vi "RH vector map_two devices_BF_LD-400_MFLI_MF-MD_PK_V5.0.vi"() -> ()   [LabVIEW 2016]
uses:
  Labview Drivers/MFLI/LabOneLabVIEW-19.05.64471/LabOneLabVIEW-19.05.64471/Zurich Instruments LabOne/Public/Configure/ziGetValueDemodSampleEx.vi
  Labview Drivers/MFLI/LabOneLabVIEW-19.05.64471/LabOneLabVIEW-19.05.64471/Zurich Instruments LabOne/Zurich Instruments LabOne.lvlib
panel:
  in  "Number average":i32=50
  out "Sweeping Magnetic Field (T)":dbl=3.018e-06 format="%#_13g"
  in  "Sweeping Magnet ramp rate (T/min)":string="0.03"
  in  "Sweeping Magnet IP Address":string="169.254.239.127"
  in  "Sweeping Magnet stabilization time (s)":dbl=1.0
  in  "From 1":dbl[](array[numeric])=[0.0] min=-3000.0 max=3000.0 format="%.1e"
  in  "To 1":dbl[](array[numeric])=[7.0] min=-3000.0 max=3000.0 format="%.1e"
  in  "Step 1":dbl[](array[numeric])=[0.05] min=-3000.0 max=3000.0 format="%.1e"
  in  "Stable Magnet stabilization time (s)":dbl=2.0 format="%#_13g"
  in  "Stable Magnet ramp rate (T/min)":string="0.03"
  out "data 2":dbl[](array[numeric])=[-1.3078e-05, 151.2, -2.85209836e-06, 4.947488930549757e-09, 8.074867339038734e-08, 16.321142810806588, -0.15000000000000074, -1.5000000000000073e-07]
  in  "Tab Control":enum32{"Device 1", "Device 2"}(tab)
  out "Rx vs H sweep (Device 1)":cluster{dbl, "Field Reading":dbl}[](graph)=[{1e-05, "Field Reading"=161.35840446232214}, {9.9e-06, "Field Reading"=41.860127097564245}, {9.800000000000001e-06, "Field Reading"=32.841407973882895}, {9.7e-06, "Field Reading"=32.83190215267119}, {9.600000000000001e-06, "Field Reading"=43.61342880349138}, {9.500000000000002e-06, "Field Reading"=37.97014058703433}, {9.400000000000001e-06, "Field Reading"=38.51287388600995}, {9.300000000000002e-06, "Field Reading"=35.71104185616921}, {9.200000000000003e-06, "Field Reading"=27.88224302316775}, {9.100000000000003e-06, "Field Reading"=31.112497747096224}, {9.000000000000004e-06, "Field Reading"=43.297646700361845}, {8.900000000000005e-06, "Field Reading"=40.66271846445741}, {8.800000000000004e-06, "Field Reading"=29.818940517533726}, {8.700000000000005e-06, "Field Reading"=31.775513272715916}, {8.600000000000006e-06, "Field Reading"=37.91978142458641}, {8.500000000000005e-06, "Field Reading"=36.71319882227341}, {8.400000000000006e-06, "Field Reading"=31.958807556261263}, {8.300000000000005e-06, "Field Reading"=43.39712342184189}, {8.200000000000006e-06, "Field Reading"=32.202863280072044}, {8.100000000000007e-06, "Field Reading"=36.33973788345392}, {8.000000000000006e-06, "Field Reading"=39.998122128750744}, {7.900000000000007e-06, "Field Reading"=42.39197863784701}, {7.800000000000008e-06, "Field Reading"=36.855072728087}, {7.700000000000008e-06, "Field Reading"=37.128132172992295}, {7.6000000000000085e-06, "Field Reading"=39.17166376756487}, {7.500000000000009e-06, "Field Reading"=39.80265360388928}, {7.40000000000001e-06, "Field Reading"=35.051759054439025}, {7.30000000000001e-06, "Field Reading"=39.481888206274185}, {7.20000000000001e-06, "Field Reading"=32.72055016297702}, {7.10000000000001e-06, "Field Reading"=28.557051745816146}, {7.000000000000011e-06, "Field Reading"=43.331293404541874}, {6.900000000000011e-06, "Field Reading"=35.81893185166727}, {6.800000000000011e-06, "Field Reading"=35.072778559533276}, {6.700000000000012e-06, "Field Reading"=35.44203632589805}, {6.600000000000012e-06, "Field Reading"=42.36422061997487}, {6.500000000000012e-06, "Field Reading"=42.01793319760923}, {6.400000000000012e-06, "Field Reading"=39.81979223345381}, {6.300000000000013e-06, "Field Reading"=45.67249265404195}, {6.2000000000000135e-06, "Field Reading"=39.54411342959387}, {6.100000000000014e-06, "Field Reading"=40.504490195623234}, {6.0000000000000146e-06, "Field Reading"=41.75691081353343}, {5.900000000000015e-06, "Field Reading"=41.452122749226305}, {5.800000000000015e-06, "Field Reading"=32.38970051842595}, {5.700000000000015e-06, "Field Reading"=43.00244438430981}, {5.600000000000016e-06, "Field Reading"=51.65721457657372}, {5.500000000000016e-06, "Field Reading"=45.63355271030433}, {5.400000000000016e-06, "Field Reading"=45.93782542419175}, {5.300000000000017e-06, "Field Reading"=45.55193121698807}, {5.200000000000017e-06, "Field Reading"=49.74200540752808}, {5.100000000000017e-06, "Field Reading"=48.779849266236944}, {5.000000000000017e-06, "Field Reading"=55.987007769383574}, {4.900000000000018e-06, "Field Reading"=49.48719028405444}, {4.800000000000018e-06, "Field Reading"=41.40308707863719}, {4.7000000000000185e-06, "Field Reading"=53.784373814286994}, {4.6000000000000195e-06, "Field Reading"=44.085575612549306}, {4.50000000000002e-06, "Field Reading"=49.718341348618466}, {4.40000000000002e-06, "Field Reading"=53.65171728330762}, {4.300000000000021e-06, "Field Reading"=59.641548125735824}, {4.200000000000021e-06, "Field Reading"=47.06243760711321}, {4.100000000000021e-06, "Field Reading"=55.39894693411911}, {4.000000000000021e-06, "Field Reading"=62.51571936174172}, {3.900000000000021e-06, "Field Reading"=68.9035008907534}, {3.8000000000000212e-06, "Field Reading"=63.99606775314202}, {3.700000000000021e-06, "Field Reading"=66.77234365785664}, {3.600000000000021e-06, "Field Reading"=69.5179299545508}, {3.5000000000000207e-06, "Field Reading"=62.954254580455874}, {3.400000000000021e-06, "Field Reading"=73.81293930429145}, {3.3000000000000205e-06, "Field Reading"=70.82103242823298}, {3.2000000000000206e-06, "Field Reading"=69.76720206210479}, {3.1000000000000207e-06, "Field Reading"=78.80471547799624}, {3.0000000000000204e-06, "Field Reading"=67.44386101206055}, {2.9000000000000205e-06, "Field Reading"=82.59912131166654}, {2.80000000000002e-06, "Field Reading"=81.12168427698563}, {2.7000000000000203e-06, "Field Reading"=81.13823856191323}, {2.60000000000002e-06, "Field Reading"=84.63690509367076}, {2.50000000000002e-06, "Field Reading"=83.00020269365744}, {2.40000000000002e-06, "Field Reading"=93.0262013428328}, {2.30000000000002e-06, "Field Reading"=91.86498911211211}, {2.2000000000000196e-06, "Field Reading"=95.78189064219018}, {2.1000000000000197e-06, "Field Reading"=97.67903895306458}, {2.0000000000000194e-06, "Field Reading"=106.0177258797565}, {1.9000000000000195e-06, "Field Reading"=112.14543741308948}, {1.8000000000000194e-06, "Field Reading"=117.94072002587943}, {1.7000000000000193e-06, "Field Reading"=128.50868647129005}, {1.6000000000000192e-06, "Field Reading"=130.73283750941107}, {1.500000000000019e-06, "Field Reading"=131.1900544205175}, {1.400000000000019e-06, "Field Reading"=136.76914635961774}, {1.3000000000000189e-06, "Field Reading"=146.35130253331926}, {1.2000000000000188e-06, "Field Reading"=159.2235400585063}, {1.1000000000000187e-06, "Field Reading"=162.39683572656568}, {1.0000000000000186e-06, "Field Reading"=183.24820207539153}, {9.000000000000187e-07, "Field Reading"=198.59616773730164}, {8.000000000000187e-07, "Field Reading"=202.29711475013792}, {7.000000000000187e-07, "Field Reading"=229.13939118910707}, {6.000000000000187e-07, "Field Reading"=352.4121711509943}, {5.000000000000187e-07, "Field Reading"=497.13445785563255}, {4.000000000000188e-07, "Field Reading"=969.1807249612372}, {3.0000000000001883e-07, "Field Reading"=2319.3065167116256}, {2.000000000000188e-07, "Field Reading"=349.016889238513}, {1.000000000000188e-07, "Field Reading"=25.587807905491125}, {1.8790524691780774e-20, "Field Reading"=15.950426066262958}, {-9.999999999998122e-08, "Field Reading"=14.841961476733772}, {-1.9999999999998122e-07, "Field Reading"=11.215795144009844}, {-2.9999999999998125e-07, "Field Reading"=8.869104703440923}, {-3.9999999999998124e-07, "Field Reading"=16.959841129659424}, {-4.999999999999812e-07, "Field Reading"=9.789433803826673}, {-5.999999999999812e-07, "Field Reading"=15.811405982830719}, {-6.999999999999812e-07, "Field Reading"=13.778561448799387}, {-7.999999999999812e-07, "Field Reading"=17.07939251134803}, {-8.999999999999811e-07, "Field Reading"=11.567482110630706}, {-9.999999999999811e-07, "Field Reading"=17.189724606732675}, {-1.0999999999999812e-06, "Field Reading"=8.534332836325326}, {-1.1999999999999813e-06, "Field Reading"=9.679059096554875}, {-1.2999999999999814e-06, "Field Reading"=19.417316586661677}, {-1.3999999999999815e-06, "Field Reading"=12.522271815596387}, {-1.4999999999999816e-06, "Field Reading"=10.165331935185511}, {-1.5999999999999817e-06, "Field Reading"=15.941613676936976}]
  out "Ix 1 (A)":dbl=1.9993378263160822e-08
  out "Vx 1 (V)":dbl=3.18726712368179e-07
  out "Rx 1 (ohm)":dbl=15.941613676936976
  in  "MFLI Device 1 Address":string="DEV4382"
  in  "File Name Device 1":string="037_S4.5_NBVJ02_dVdImapping(Bz)_I18_R45_ac20nA(7.919Hz)_dcpre1_range0.2_step1.5m"
  out "Vy 1 (V)":dbl format="%#_13g"
  out "Iy 1 (A)":dbl format="%#_13g"
  in  "Folder":path=path "D:/Heng/Nb3Br8_JJ/Sb.3_NBVJ01"
  in  "MFLI Device 2 Address":string="DEV4496"
  in  "File Name Device 2":string="037_Sb.3_NBVJ01_dVdI_mapping(Bz)_I16_R34_ac5nA(13.3337Hz)_dcpre1_range0.2_step1.5m"
  out "Rx vs H sweep (Device 2)":cluster{dbl, "Field Reading":dbl}[](graph)=[{1e-05, "Field Reading"=161.35840446232214}, {9.9e-06, "Field Reading"=41.860127097564245}, {9.800000000000001e-06, "Field Reading"=32.841407973882895}, {9.7e-06, "Field Reading"=32.83190215267119}, {9.600000000000001e-06, "Field Reading"=43.61342880349138}, {9.500000000000002e-06, "Field Reading"=37.97014058703433}, {9.400000000000001e-06, "Field Reading"=38.51287388600995}, {9.300000000000002e-06, "Field Reading"=35.71104185616921}, {9.200000000000003e-06, "Field Reading"=27.88224302316775}, {9.100000000000003e-06, "Field Reading"=31.112497747096224}, {9.000000000000004e-06, "Field Reading"=43.297646700361845}, {8.900000000000005e-06, "Field Reading"=40.66271846445741}, {8.800000000000004e-06, "Field Reading"=29.818940517533726}, {8.700000000000005e-06, "Field Reading"=31.775513272715916}, {8.600000000000006e-06, "Field Reading"=37.91978142458641}, {8.500000000000005e-06, "Field Reading"=36.71319882227341}, {8.400000000000006e-06, "Field Reading"=31.958807556261263}, {8.300000000000005e-06, "Field Reading"=43.39712342184189}, {8.200000000000006e-06, "Field Reading"=32.202863280072044}, {8.100000000000007e-06, "Field Reading"=36.33973788345392}, {8.000000000000006e-06, "Field Reading"=39.998122128750744}, {7.900000000000007e-06, "Field Reading"=42.39197863784701}, {7.800000000000008e-06, "Field Reading"=36.855072728087}, {7.700000000000008e-06, "Field Reading"=37.128132172992295}, {7.6000000000000085e-06, "Field Reading"=39.17166376756487}, {7.500000000000009e-06, "Field Reading"=39.80265360388928}, {7.40000000000001e-06, "Field Reading"=35.051759054439025}, {7.30000000000001e-06, "Field Reading"=39.481888206274185}, {7.20000000000001e-06, "Field Reading"=32.72055016297702}, {7.10000000000001e-06, "Field Reading"=28.557051745816146}, {7.000000000000011e-06, "Field Reading"=43.331293404541874}, {6.900000000000011e-06, "Field Reading"=35.81893185166727}, {6.800000000000011e-06, "Field Reading"=35.072778559533276}, {6.700000000000012e-06, "Field Reading"=35.44203632589805}, {6.600000000000012e-06, "Field Reading"=42.36422061997487}, {6.500000000000012e-06, "Field Reading"=42.01793319760923}, {6.400000000000012e-06, "Field Reading"=39.81979223345381}, {6.300000000000013e-06, "Field Reading"=45.67249265404195}, {6.2000000000000135e-06, "Field Reading"=39.54411342959387}, {6.100000000000014e-06, "Field Reading"=40.504490195623234}, {6.0000000000000146e-06, "Field Reading"=41.75691081353343}, {5.900000000000015e-06, "Field Reading"=41.452122749226305}, {5.800000000000015e-06, "Field Reading"=32.38970051842595}, {5.700000000000015e-06, "Field Reading"=43.00244438430981}, {5.600000000000016e-06, "Field Reading"=51.65721457657372}, {5.500000000000016e-06, "Field Reading"=45.63355271030433}, {5.400000000000016e-06, "Field Reading"=45.93782542419175}, {5.300000000000017e-06, "Field Reading"=45.55193121698807}, {5.200000000000017e-06, "Field Reading"=49.74200540752808}, {5.100000000000017e-06, "Field Reading"=48.779849266236944}, {5.000000000000017e-06, "Field Reading"=55.987007769383574}, {4.900000000000018e-06, "Field Reading"=49.48719028405444}, {4.800000000000018e-06, "Field Reading"=41.40308707863719}, {4.7000000000000185e-06, "Field Reading"=53.784373814286994}, {4.6000000000000195e-06, "Field Reading"=44.085575612549306}, {4.50000000000002e-06, "Field Reading"=49.718341348618466}, {4.40000000000002e-06, "Field Reading"=53.65171728330762}, {4.300000000000021e-06, "Field Reading"=59.641548125735824}, {4.200000000000021e-06, "Field Reading"=47.06243760711321}, {4.100000000000021e-06, "Field Reading"=55.39894693411911}, {4.000000000000021e-06, "Field Reading"=62.51571936174172}, {3.900000000000021e-06, "Field Reading"=68.9035008907534}, {3.8000000000000212e-06, "Field Reading"=63.99606775314202}, {3.700000000000021e-06, "Field Reading"=66.77234365785664}, {3.600000000000021e-06, "Field Reading"=69.5179299545508}, {3.5000000000000207e-06, "Field Reading"=62.954254580455874}, {3.400000000000021e-06, "Field Reading"=73.81293930429145}, {3.3000000000000205e-06, "Field Reading"=70.82103242823298}, {3.2000000000000206e-06, "Field Reading"=69.76720206210479}, {3.1000000000000207e-06, "Field Reading"=78.80471547799624}, {3.0000000000000204e-06, "Field Reading"=67.44386101206055}, {2.9000000000000205e-06, "Field Reading"=82.59912131166654}, {2.80000000000002e-06, "Field Reading"=81.12168427698563}, {2.7000000000000203e-06, "Field Reading"=81.13823856191323}, {2.60000000000002e-06, "Field Reading"=84.63690509367076}, {2.50000000000002e-06, "Field Reading"=83.00020269365744}, {2.40000000000002e-06, "Field Reading"=93.0262013428328}, {2.30000000000002e-06, "Field Reading"=91.86498911211211}, {2.2000000000000196e-06, "Field Reading"=95.78189064219018}, {2.1000000000000197e-06, "Field Reading"=97.67903895306458}, {2.0000000000000194e-06, "Field Reading"=106.0177258797565}, {1.9000000000000195e-06, "Field Reading"=112.14543741308948}, {1.8000000000000194e-06, "Field Reading"=117.94072002587943}, {1.7000000000000193e-06, "Field Reading"=128.50868647129005}, {1.6000000000000192e-06, "Field Reading"=130.73283750941107}, {1.500000000000019e-06, "Field Reading"=131.1900544205175}, {1.400000000000019e-06, "Field Reading"=136.76914635961774}, {1.3000000000000189e-06, "Field Reading"=146.35130253331926}, {1.2000000000000188e-06, "Field Reading"=159.2235400585063}, {1.1000000000000187e-06, "Field Reading"=162.39683572656568}, {1.0000000000000186e-06, "Field Reading"=183.24820207539153}, {9.000000000000187e-07, "Field Reading"=198.59616773730164}, {8.000000000000187e-07, "Field Reading"=202.29711475013792}, {7.000000000000187e-07, "Field Reading"=229.13939118910707}, {6.000000000000187e-07, "Field Reading"=352.4121711509943}, {5.000000000000187e-07, "Field Reading"=497.13445785563255}, {4.000000000000188e-07, "Field Reading"=969.1807249612372}, {3.0000000000001883e-07, "Field Reading"=2319.3065167116256}, {2.000000000000188e-07, "Field Reading"=349.016889238513}, {1.000000000000188e-07, "Field Reading"=25.587807905491125}, {1.8790524691780774e-20, "Field Reading"=15.950426066262958}, {-9.999999999998122e-08, "Field Reading"=14.841961476733772}, {-1.9999999999998122e-07, "Field Reading"=11.215795144009844}, {-2.9999999999998125e-07, "Field Reading"=8.869104703440923}, {-3.9999999999998124e-07, "Field Reading"=16.959841129659424}, {-4.999999999999812e-07, "Field Reading"=9.789433803826673}, {-5.999999999999812e-07, "Field Reading"=15.811405982830719}, {-6.999999999999812e-07, "Field Reading"=13.778561448799387}, {-7.999999999999812e-07, "Field Reading"=17.07939251134803}, {-8.999999999999811e-07, "Field Reading"=11.567482110630706}, {-9.999999999999811e-07, "Field Reading"=17.189724606732675}, {-1.0999999999999812e-06, "Field Reading"=8.534332836325326}, {-1.1999999999999813e-06, "Field Reading"=9.679059096554875}, {-1.2999999999999814e-06, "Field Reading"=19.417316586661677}, {-1.3999999999999815e-06, "Field Reading"=12.522271815596387}, {-1.4999999999999816e-06, "Field Reading"=10.165331935185511}, {-1.5999999999999817e-06, "Field Reading"=15.941613676936976}]
  out "Vx 2 (V)":dbl format="%#_13g"
  out "Vy 2 (V)":dbl format="%#_13g"
  out "Ix 2 (A)":dbl format="%#_13g"
  out "Iy 2 (A)":dbl format="%#_13g"
  out "Rx 2 (ohm)":dbl=15.941613676936976
  in  "Folder 2":path=path "D:/Heng/Nb3Br8_JJ/Sb.3_NBVJ01"
  out "File path 2":path=path "D:/Heng/Nb3Br8_JJ/Sb.3_NBVJ01/034_Sb.3_NBVJ01_dVdI_mapping(Bz)_I16_R34_ac5nA(13.3337Hz)_dcpre1_range0.2_step1.5m.dat"
  in  "Step":dbl[](array[numeric])=[0.0015] min=-3000.0 max=3000.0 format="%.1e"
  in  "To":dbl[](array[numeric])=[0.0] min=-3000.0 max=3000.0 format="%.1e"
  in  "From":dbl[](array[numeric])=[0.0] min=-3000.0 max=3000.0 format="%.1e"
  in  "Stable Magnet IP Address":string="169.254.239.127"
  out "Stable Magnetic Field (T)":dbl=3.018e-06 format="%#_13g"
  in  "stop":bool
  out "Time (s)":dbl=155.767
  out "data":dbl[](array[numeric])=[3.018e-06, 155.767, -2.52078936e-06, 1.9993378263160822e-08, 3.18726712368179e-07, 15.941613676936976, -0.7999999999999908, -1.5999999999999817e-06]
  out "File path 1":path=path "D:/Heng/Nb3Br8_JJ/Sb.3_NBVJ01/034_S4.5_NBVJ02_dVdImapping(Bz)_I18_R45_ac20nA(7.919Hz)_dcpre1_range0.2_step1.5m.dat"
  # "Set Stable  Magnetic Field (T)"
  # "Set  Sweeping Magnetic field (T)"
  # ".dat"
  # ".dat"
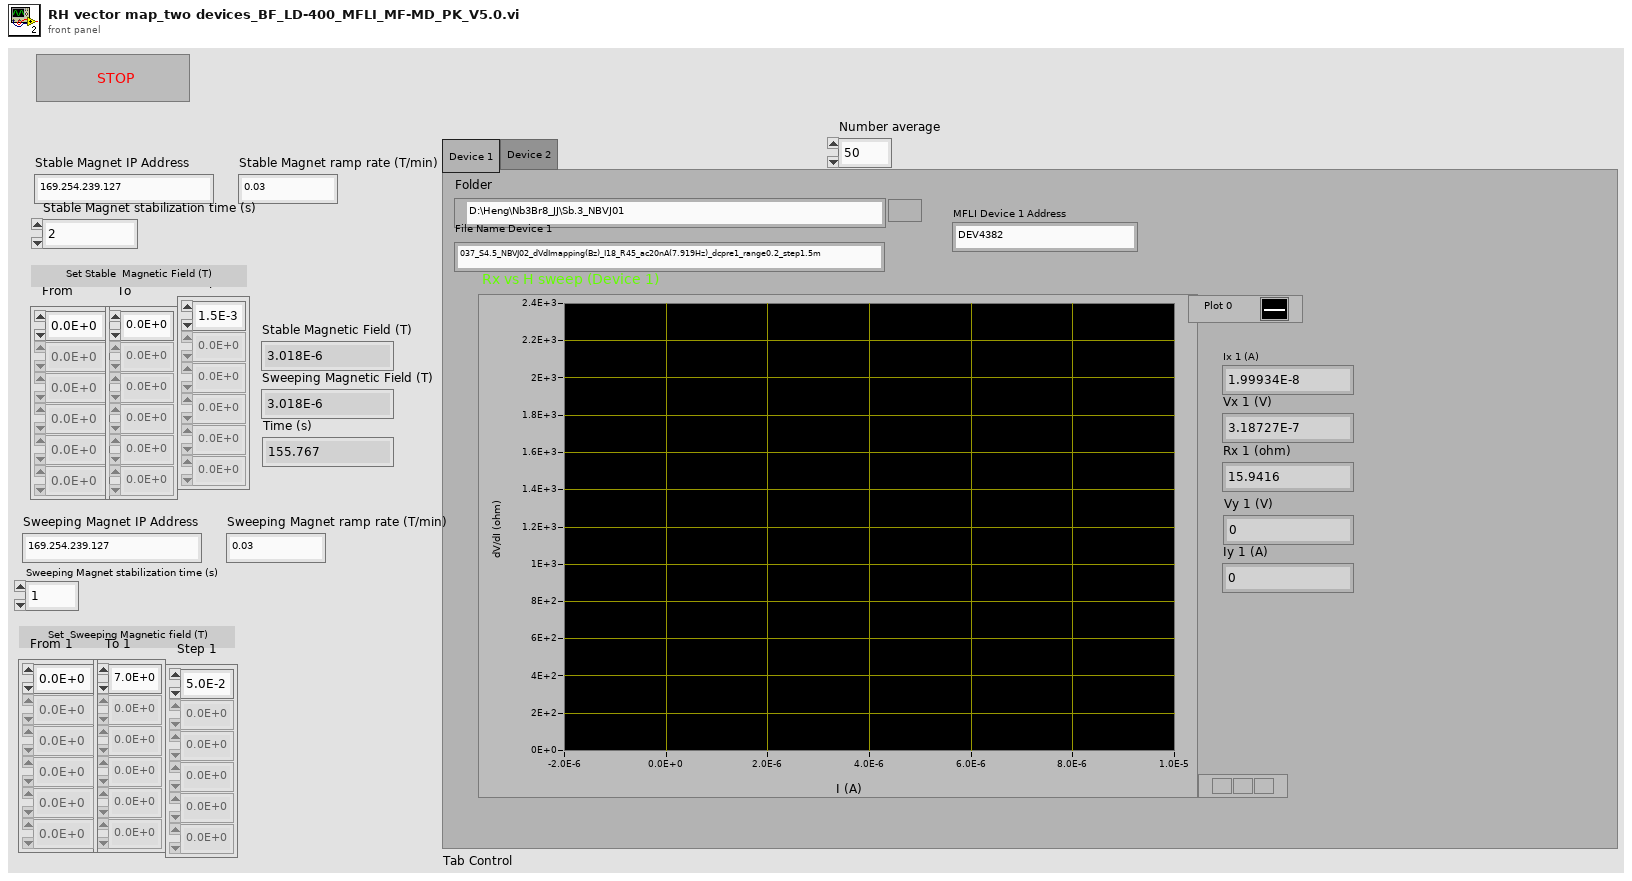
[diagram p1: front panel]
types:
  T1 = enum16{"open", "replace", "create", "open or create", "replace or create", "replace or create with confirmation"}
  T2 = typedef "Zurich Instruments LabOne.lvlib/ziTypeHandle.ctl" = cluster{"handleValid":bool, "Conn":u64, "Path Prefix":string, "Handle":u64, "Connected":bool, "Clockbase(s)":dbl}
  T3 = typedef "Zurich Instruments LabOne.lvlib/ziTypeDemodSampleSingle.ctl" = cluster{"Timestamps (ticks)":u64, "X (Vrms)":dbl, "Y (Vrms)":dbl, "Osc Phase (deg)":dbl, "Freq (Hz)":dbl, "DIO":u32, "AuxIn0 (V)":dbl, "AuxIn1 (V)":dbl, "Trigger":u32}
  T4 = cluster{"Sweeping Magnetic Field (T)":dbl, "Field Reading":dbl}[]
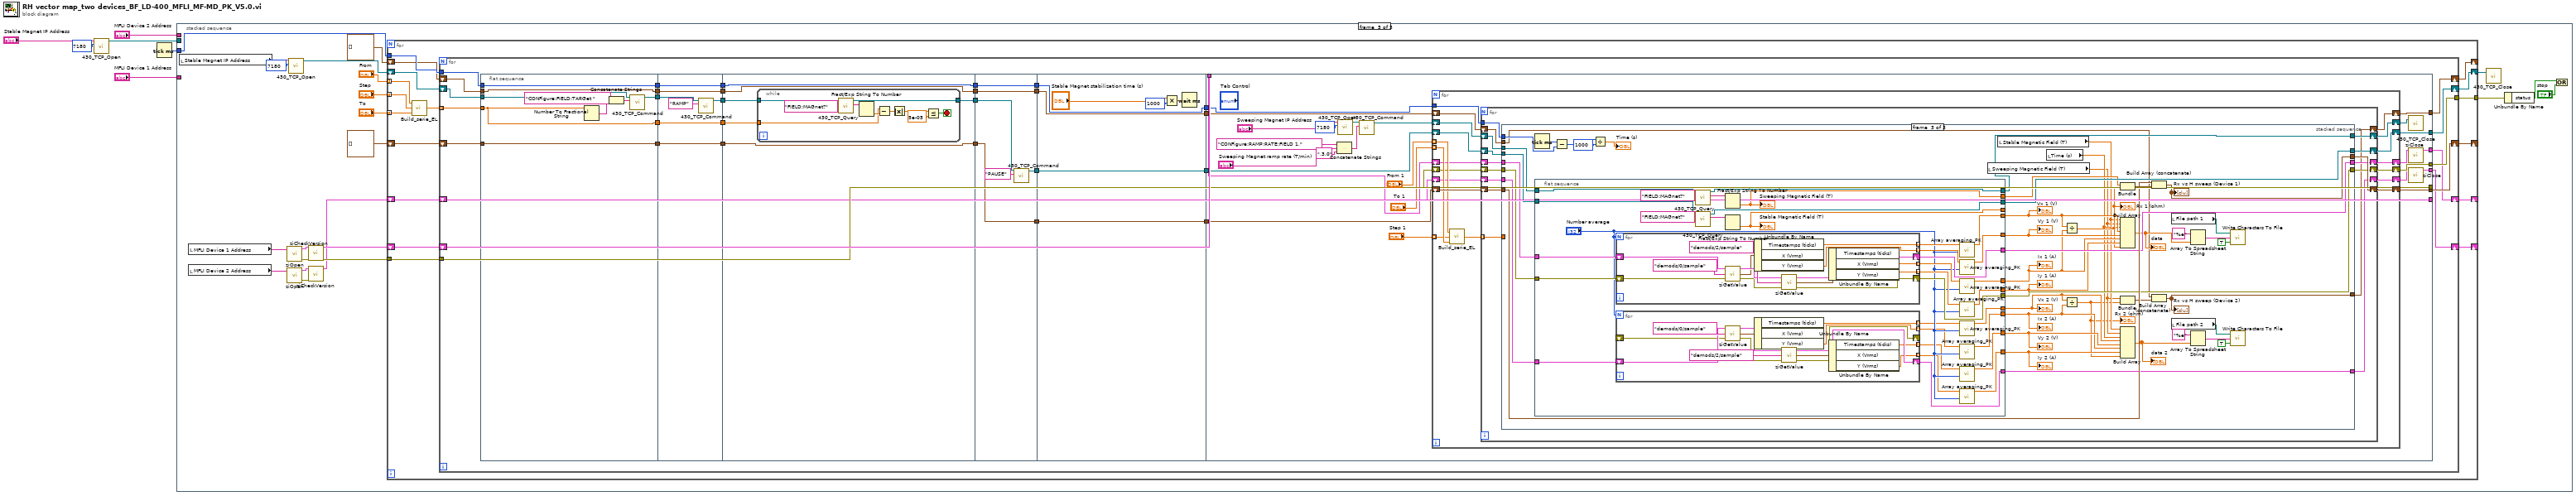
[diagram p0: block diagram]
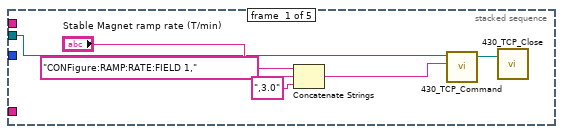
[diagram p2: hidden frame]
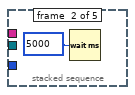
[diagram p3: hidden frame]
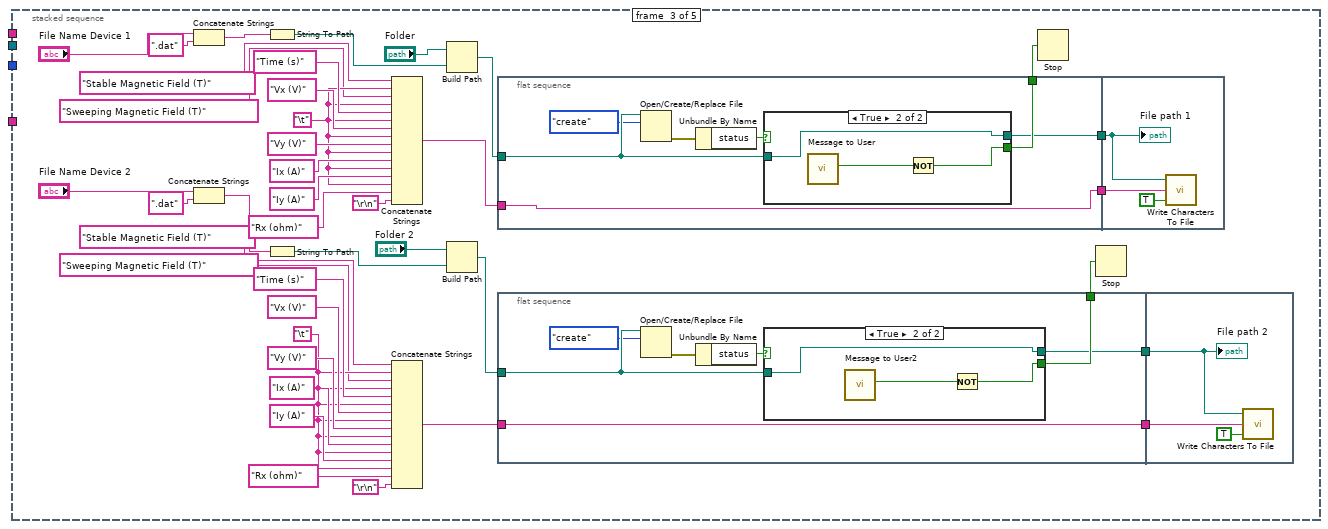
[diagram p4: hidden frame]
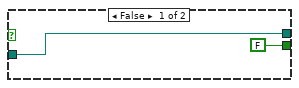
[diagram p5: hidden frame]
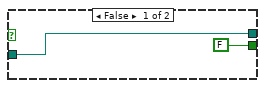
[diagram p6: hidden frame]
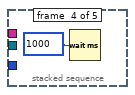
[diagram p7: hidden frame]
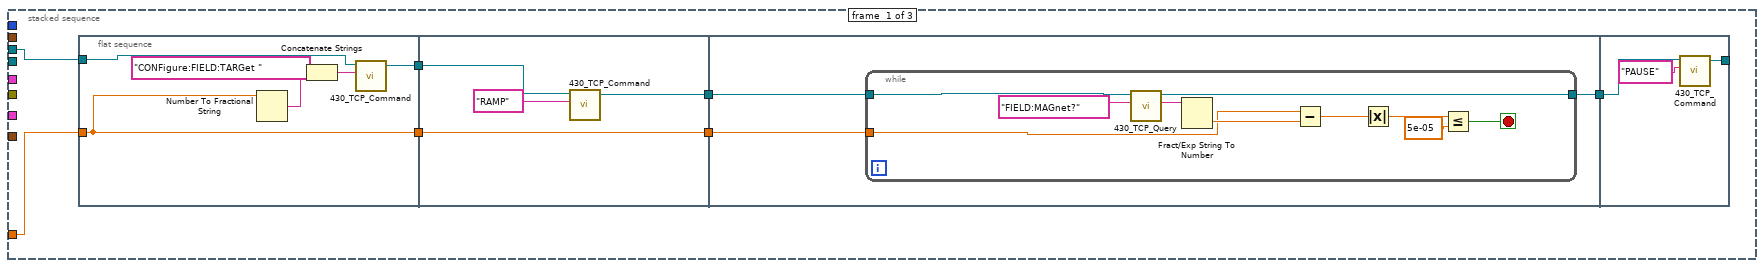
[diagram p8: hidden frame]
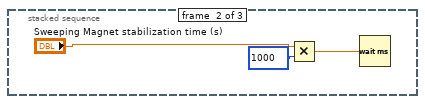
[diagram p9: hidden frame]
diagram:
  n1 = call "430_TCP_Open.vi"("IP Address"="Stable Magnet IP Address", "TCP Port"=7180) -> ("connection ID"=w2:refnum<k5>)  [unwired: 4 in, 2 out]
  n2 = Tick Count (ms)() -> (millisecond timer value=w5:u32)
  n3 = stacked-sequence {
    tunnel: "MFLI Device 1 Address" -> [_ _ _ _ _]
    tunnel: w5 -> [_ _ _ _ w105]
    tunnel: w2 -> [w7 _ _ _ _]
    tunnel: "MFLI Device 2 Address" -> [_ _ _ _ _]
    frame #0 {
      n4 = Concatenate Strings("CONFigure:RAMP:RATE:FIELD 1," ("String"), "Stable Magnet ramp rate (T/min)", ",3.0") -> (w8:string)
      n5 = call "430_TCP_Command.vi"("Command"=w8, "connection ID"=w7) -> ("connection ID out"=w12:refnum<k5>)  [unwired: 2 in, 2 out]
      n6 = call "430_TCP_Close.vi"("connection ID"=w12) -> ()  [unwired: 1 in, 2 out]
    }
    frame #1 {
      n7 = Wait (ms)(milliseconds to wait=5000) -> ()  [unwired: 1 out]
    }
    frame #2 {
      w16 = "\t"
      w26 = "\t"
      n8 = Concatenate Strings("File Name Device 1", ".dat" ("string")) -> (w50:string)
      n9 = Concatenate Strings("File Name Device 2", ".dat" ("string")) -> (w33:string)
      n10 = String To Path(string=w50) -> (path=w42:path)
      n11 = String To Path(string=w33) -> (path=w30:path)
      n12 = Concatenate Strings("Stable Magnetic Field (T)", w26, "Sweeping Magnetic Field (T)", w26, "Time (s)", w26, "Vx (V)" ("string"), w26, "Vy (V)" ("string"), w26, "Ix (A)" ("string"), w26, "Iy (A)", w26, "Rx (ohm)", "\r\n") -> (w51:string)
      n13 = Concatenate Strings("Stable Magnetic Field (T)", w16, "Sweeping Magnetic Field (T)", w16, "Time (s)", w16, "Vx (V)" ("string"), w16, "Vy (V)" ("string"), w16, "Ix (A)" ("string"), w16, "Iy (A)", w16, "Rx (ohm)", "\r\n") -> (w14:string)
      n14 = Build Path(base path="Folder", name or relative path=w42) -> (appended path=w41:path)
      n15 = Build Path(base path="Folder 2", name or relative path=w30) -> (appended path=w29:path)
      n16 = flat-sequence {
        tunnel: w41 -> [w72]
        tunnel: w51 -> [w75]
        tunnel: [w75] -> w53
        tunnel: [w74] -> w48
        tunnel: [w73] -> w52
        tunnel: w53 -> [w82]
        tunnel: w52 -> [w81]
        frame #0 {
          n17 = Open/Create/Replace File(file path (use dialog)=w72, operation (0:open)=T1."create") -> (error out=w71:errorcluster)  [unwired: 4 in, 2 out]
          n18 = Unbundle By Name(w71) -> ("status"=w69:bool)
          n19 = case shown="True" w69 {
            tunnel: [FALSE ("Yes") w79] -> w74
            tunnel: [w76 w78] -> w73
            tunnel: w72 -> [w76 w78]
            frame False {
            }
            frame True {
              n20 = call "Message to User"() -> ("Yes"=w80:bool)  [unwired: 10 in, 1 out]
              n21 = Not(x=w80) -> (.not. x?=w79:bool)
            }
          }
        }
        frame #1 {
          n22 = call <vilib>:"Write Characters To File.vi"("append to file? (new file:F)"=TRUE, "character string"=w82, "file path (dialog if empty)"=w81) -> ()  [unwired: 2 in, 1 out]
          "File path 1" <- w81
        }
      }
      n23 = flat-sequence {
        tunnel: w29 -> [w57]
        tunnel: w14 -> [w60]
        tunnel: [w60] -> w35
        tunnel: [w59] -> w32
        tunnel: [w58] -> w34
        tunnel: w35 -> [w67]
        tunnel: w34 -> [w66]
        frame #0 {
          n24 = Open/Create/Replace File(file path (use dialog)=w57, operation (0:open)=T1."create") -> (error out=w56:errorcluster)  [unwired: 4 in, 2 out]
          n25 = Unbundle By Name(w56) -> ("status"=w54:bool)
          n26 = case shown="True" w54 {
            tunnel: [FALSE ("Yes") w64] -> w59
            tunnel: [w61 w63] -> w58
            tunnel: w57 -> [w61 w63]
            frame False {
            }
            frame True {
              n27 = call "Message to User2"() -> ("Yes"=w65:bool)  [unwired: 10 in, 1 out]
              n28 = Not(x=w65) -> (.not. x?=w64:bool)
            }
          }
        }
        frame #1 {
          n29 = call <vilib>:"Write Characters To File.vi"("append to file? (new file:F)"=TRUE, "character string"=w67, "file path (dialog if empty)"=w66) -> ()  [unwired: 2 in, 1 out]
          "File path 2" <- w66
        }
      }
      n30 = Stop(stop? (T)=w48) -> ()
      n31 = Stop(stop? (T)=w32) -> ()
    }
    frame #3 {
      n32 = Wait (ms)(milliseconds to wait=u32 1000) -> ()  [unwired: 1 out]
    }
    frame #4 {
      n33 = local read "Stable Magnet IP Address"() -> (w95:string)
      n34 = local read "MFLI Device 1 Address"() -> (w92:string)
      n35 = local read "MFLI Device 2 Address"() -> (w89:string)
      n36 = call "ziOpen.vi"("Address"=w92) -> ("Error Out"=w91:errorcluster, "HandleOut"=w93:T2)  [unwired: 3 in, 1 out]
      n37 = call "ziOpen.vi"("Address"=w89) -> ("Error Out"=w88:errorcluster, "HandleOut"=w90:T2)  [unwired: 3 in, 1 out]
      n38 = call "430_TCP_Open.vi"("IP Address"=w95, "TCP Port"=7180) -> ("connection ID"=w94:refnum<k5>)  [unwired: 4 in, 2 out]
      n39 = call "ziCheckVersion.vi"("Handle In"=w93, "Error In"=w91) -> ("Handle Out"=w87:T2, "Error Out"=w86:errorcluster)  [unwired: 11 in, 1 out]
      n40 = call "ziCheckVersion.vi"("Handle In"=w90, "Error In"=w88) -> ("Handle Out"=w85:T2)  [unwired: 11 in, 2 out]
      n41 = for {
        tunnel: w105 -> [w122]
        tunnel: "From" -> [w121] mode=indexing
        tunnel: "Step" -> [w120] mode=indexing
        tunnel: "To" -> [w119] mode=indexing
        shift-right: [w118] -> _
        shift-left: cluster{dbl, "Field Reading":dbl}[] [] -> [w123]
        tunnel: [w116] -> w100
        shift-right: [w115] -> _
        shift-left: cluster{dbl, "Field Reading":dbl}[] [] -> [w114]
        shift-right: [w113] -> w97
        shift-left: w94 -> [w112]
        tunnel: w86 -> [w110]
        shift-right: [w108] -> _
        shift-left: w85 -> [w109]
        shift-right: [w107] -> _
        shift-left: w87 -> [w111]
        n42 = call "Build_serie_EL.vi"("end value"=w119, "increment"=w120, "start value"=w121) -> ("output array"=w117:dbl[])
        n43 = for {
          tunnel: w122 -> [w152]
          shift-right: [w151] -> w118
          shift-left: w123 -> [w153]
          tunnel: w117 -> [w150] mode=indexing
          tunnel: [w144] -> w116
          shift-right: [w129] -> w115
          shift-left: w114 -> [w140]
          shift-right: [w139] -> w113
          shift-left: w112 -> [w138]
          tunnel: w110 -> [w127]
          shift-right: [w125] -> w108
          shift-left: w109 -> [w126]
          shift-right: [w124] -> w107
          shift-left: w111 -> [w128]
          n44 = flat-sequence {
            tunnel: w152 -> [w167]
            tunnel: w153 -> [w168]
            tunnel: [w168] -> w159
            tunnel: [w167] -> w158
            tunnel: w150 -> [w162]
            tunnel: [w163] -> w149
            tunnel: [w162] -> w146
            tunnel: [w161] -> w143
            tunnel: w140 -> [w161]
            tunnel: w138 -> [w160]
            tunnel: [w175] -> w157
            tunnel: [w174] -> w156
            tunnel: w159 -> [w175]
            tunnel: w158 -> [w174]
            tunnel: w149 -> [w172]
            tunnel: [w171] -> w148
            tunnel: [w170] -> w147
            tunnel: w146 -> [w170]
            tunnel: w143 -> [w169]
            tunnel: [w169] -> w142
            tunnel: [w181] -> w137
            tunnel: [w180] -> w135
            tunnel: w157 -> [w181]
            tunnel: w156 -> [w180]
            tunnel: w148 -> [w179]
            tunnel: w147 -> [w178]
            tunnel: [w177] -> w133
            tunnel: w142 -> [w176]
            tunnel: [w176] -> w131
            tunnel: w137 -> [w197]
            tunnel: [w197] -> w136
            tunnel: w135 -> [w196]
            tunnel: [w196] -> w134
            tunnel: w133 -> [w193]
            tunnel: [w192] -> w132
            tunnel: w131 -> [w195]
            tunnel: [w195] -> w130
            tunnel: [w204] -> w155
            tunnel: [w203] -> w154
            tunnel: w136 -> [w204]
            tunnel: w134 -> [w203]
            tunnel: [w199] -> w145
            tunnel: w132 -> [w199]
            tunnel: w130 -> [w198]
            tunnel: [w198] -> w141
            tunnel: [w226] -> w144
            tunnel: w155 -> [w228]
            tunnel: w154 -> [w227]
            tunnel: [w225] -> w151
            tunnel: w145 -> [w224]
            tunnel: w141 -> [w210]
            tunnel: [w220] -> w139
            tunnel: [w211] -> w129
            tunnel: w128 -> [w209]
            tunnel: w127 -> [w208]
            tunnel: w126 -> [w207]
            tunnel: [w206] -> w125
            tunnel: [w205] -> w124
            frame #0 {
              n45 = Number To Fractional String(number=w162) -> (F-format string=w164:string)  [unwired: 3 in]
              n46 = Concatenate Strings("CONFigure:FIELD:TARGet " ("String"), w164) -> (w166:string)
              n47 = call "430_TCP_Command.vi"("Command"=w166, "connection ID"=w160) -> ("connection ID out"=w163:refnum<k5>)  [unwired: 2 in, 2 out]
            }
            frame #1 {
              n48 = call "430_TCP_Command.vi"("Command"="RAMP", "connection ID"=w172) -> ("connection ID out"=w171:refnum<k5>)  [unwired: 2 in, 2 out]
            }
            frame #2 {
              n49 = while {
                tunnel: w179 -> [w191]
                tunnel: w178 -> [w186]
                tunnel: [w182] -> w177
                stop <- w184 stop-if-true
                n50 = call "430_TCP_Query.vi"("Command"="FIELD:MAGnet?" ("String"), "connection ID"=w191) -> ("Response"=w190:string, "connection ID out"=w182:refnum<k5>)  [unwired: 5 in, 3 out]
                n51 = Fract/Exp String To Number(string=w190) -> (number=w187:dbl)  [unwired: 3 in, 1 out]
                n52 = Subtract(x=w186, y=w187) -> (x-y=w189:dbl)
                n53 = Absolute Value(x=w189) -> (abs(x)=w188:dbl)
                n54 = Less Or Equal?(x=w188, y=5e-05) -> (x <= y?=w184:bool)
              }
            }
            frame #3 {
              n55 = call "430_TCP_Command.vi"("Command"="PAUSE", "connection ID"=w193) -> ("connection ID out"=w192:refnum<k5>)  [unwired: 2 in, 2 out]
            }
            frame #4 {
              n56 = Multiply(x="Stable Magnet stabilization time (s)", y=1000) -> (x*y=w201:dbl)
              n57 = Wait (ms)(milliseconds to wait=w201) -> ()  [unwired: 1 out]
            }
            frame #5 {
              n58 = Concatenate Strings("CONFigure:RAMP:RATE:FIELD 1," ("String"), "Sweeping Magnet ramp rate (T/min)", ",3.0") -> (w217:string)
              n59 = call "430_TCP_Open.vi"("IP Address"="Sweeping Magnet IP Address", "TCP Port"=7180) -> ("connection ID"=w215:refnum<k5>)  [unwired: 4 in, 2 out]
              n60 = call "430_TCP_Command.vi"("Command"=w217, "connection ID"=w215) -> ("connection ID out"=w214:refnum<k5>)  [unwired: 2 in, 2 out]
              n61 = for {
                tunnel: "From 1" -> [w247] mode=indexing
                tunnel: "To 1" -> [w246] mode=indexing
                tunnel: "Step 1" -> [w245] mode=indexing
                shift-right: [w249] -> w225
                shift-left: w228 -> [w250]
                tunnel: w227 -> [w244]
                shift-right: [w242] -> w223
                shift-left: w209 -> [w243]
                shift-right: [w241] -> w226
                shift-left: w208 -> [w240]
                shift-right: [w238] -> w220
                shift-left: w224 -> [w239]
                shift-right: [w236] -> w221
                shift-left: w214 -> [w237]
                shift-right: [w234] -> w212
                shift-left: w207 -> [w235]
                shift-right: [w233] -> w211
                shift-left: w210 -> [w232]
                n62 = call "Build_serie_EL.vi"("end value"=w246, "increment"=w245, "start value"=w247) -> ("output array"=w248:dbl[])
                n63 = for {
                  tunnel: w248 -> [w266] mode=indexing
                  shift-right: [w264] -> w249
                  shift-left: w250 -> [w265]
                  tunnel: w244 -> [w263]
                  shift-right: [w261] -> w242
                  shift-left: w243 -> [w262]
                  shift-right: [w260] -> w241
                  shift-left: w240 -> [w259]
                  shift-right: [w257] -> w238
                  shift-left: w239 -> [w258]
                  shift-right: [w255] -> w236
                  shift-left: w237 -> [w256]
                  shift-right: [w253] -> w234
                  shift-left: w235 -> [w254]
                  shift-right: [w252] -> w233
                  shift-left: w232 -> [w251]
                  n64 = stacked-sequence {
                    tunnel: w265 -> [_ _ w346]
                    tunnel: w266 -> [w273 _ _]
                    tunnel: [_ _ w345] -> w264
                    tunnel: w263 -> [_ _ w343]
                    tunnel: w262 -> [_ _ w339]
                    tunnel: [_ _ w338] -> w261
                    tunnel: [_ _ w337] -> w260
                    tunnel: w259 -> [_ _ w336]
                    tunnel: w258 -> [_ _ w329]
                    tunnel: [_ _ w330] -> w257
                    tunnel: w256 -> [w272 _ w328]
                    tunnel: [_ _ w327] -> w255
                    tunnel: w254 -> [_ _ w320]
                    tunnel: [_ _ w310] -> w253
                    tunnel: [_ _ w309] -> w252
                    tunnel: w251 -> [_ _ w308]
                    frame #0 {
                      n65 = flat-sequence {
                        tunnel: w273 -> [w274]
                        tunnel: w272 -> [w276]
                        tunnel: [w275] -> w271
                        tunnel: [w274] -> w268
                        tunnel: w271 -> [w282]
                        tunnel: [w281] -> w270
                        tunnel: [w280] -> w269
                        tunnel: w268 -> [w280]
                        tunnel: w270 -> [w286]
                        tunnel: w269 -> [w285]
                        tunnel: [w284] -> w267
                        tunnel: [w298] -> _
                        tunnel: w267 -> [w297]
                        frame #0 {
                          n66 = Number To Fractional String(number=w274) -> (F-format string=w278:string)  [unwired: 3 in]
                          n67 = Concatenate Strings("CONFigure:FIELD:TARGet " ("String"), w278) -> (w277:string)
                          n68 = call "430_TCP_Command.vi"("Command"=w277, "connection ID"=w276) -> ("connection ID out"=w275:refnum<k5>)  [unwired: 2 in, 2 out]
                        }
                        frame #1 {
                          n69 = call "430_TCP_Command.vi"("Command"="RAMP", "connection ID"=w282) -> ("connection ID out"=w281:refnum<k5>)  [unwired: 2 in, 2 out]
                        }
                        frame #2 {
                          n70 = while {
                            tunnel: w286 -> [w296]
                            tunnel: w285 -> [w291]
                            tunnel: [w287] -> w284
                            stop <- w289 stop-if-true
                            n71 = call "430_TCP_Query.vi"("Command"="FIELD:MAGnet?" ("String"), "connection ID"=w296) -> ("Response"=w295:string, "connection ID out"=w287:refnum<k5>)  [unwired: 5 in, 3 out]
                            n72 = Fract/Exp String To Number(string=w295) -> (number=w292:dbl)  [unwired: 3 in, 1 out]
                            n73 = Subtract(x=w291, y=w292) -> (x-y=w294:dbl)
                            n74 = Absolute Value(x=w294) -> (abs(x)=w293:dbl)
                            n75 = Less Or Equal?(x=w293, y=5e-05) -> (x <= y?=w289:bool)
                          }
                        }
                        frame #3 {
                          n76 = call "430_TCP_Command.vi"("Command"="PAUSE", "connection ID"=w297) -> ("connection ID out"=w298:refnum<k5>)  [unwired: 2 in, 2 out]
                        }
                      }
                    }
                    frame #1 {
                      n77 = Multiply(x="Sweeping Magnet stabilization time (s)", y=1000) -> (x*y=w301:dbl)
                      n78 = Wait (ms)(milliseconds to wait=w301) -> ()  [unwired: 1 out]
                    }
                    frame #2 {
                      n79 = Tick Count (ms)() -> (millisecond timer value=w344:u32)
                      n80 = flat-sequence {
                        tunnel: [w366] -> w325
                        tunnel: [w363] -> w323
                        tunnel: [w379] -> w337
                        tunnel: [w380] -> w338
                        tunnel: [w372] -> _
                        tunnel: [w373] -> w330
                        tunnel: w329 -> [w374]
                        tunnel: w336 -> [w377]
                        tunnel: w339 -> [w378]
                        tunnel: w328 -> [w370]
                        tunnel: [w368] -> w327
                        tunnel: [w361] -> w324
                        tunnel: [w360] -> w322
                        tunnel: [w359] -> w326
                        tunnel: w320 -> [w358]
                        tunnel: [w352] -> w314
                        tunnel: [w351] -> w317
                        tunnel: [w350] -> w313
                        tunnel: [w349] -> w316
                        tunnel: [w348] -> w310
                        frame #0 {
                          n81 = for {
                            N: "Number average" -> [_]
                            tunnel: [w404] -> w364 mode=indexing
                            tunnel: [w403] -> w362 mode=indexing
                            tunnel: [w398] -> w367 mode=indexing
                            tunnel: [w397] -> w365 mode=indexing
                            shift-right: [w408] -> w380
                            shift-left: w378 -> [w396]
                            shift-right: [w407] -> w379
                            shift-left: w377 -> [w395]
                            n82 = call-poly "ziGetValue.vi"("error in"=w395, "Path"="demods/0/sample", "Handle In"=w396) -> ("error out"=w401:errorcluster, "Demod Sample Out"=w399:T3, "Handle Out"=w402:T2)
                            n83 = Unbundle By Name(w399) -> ("X (Vrms)"=w398:dbl, "Y (Vrms)"=w397:dbl)  [unwired: 1 out]
                            n84 = call-poly "ziGetValue.vi"("error in"=w401, "Path"="demods/2/sample", "Handle In"=w402) -> ("error out"=w407:errorcluster, "Demod Sample Out"=w405:T3, "Handle Out"=w408:T2)
                            n85 = Unbundle By Name(w405) -> ("X (Vrms)"=w404:dbl, "Y (Vrms)"=w403:dbl)  [unwired: 1 out]
                          }
                          n86 = for {
                            N: "Number average" -> [_]
                            tunnel: [w390] -> w355 mode=indexing
                            tunnel: [w389] -> w353 mode=indexing
                            tunnel: [w384] -> w356 mode=indexing
                            tunnel: [w383] -> w354 mode=indexing
                            shift-right: [w394] -> w348
                            shift-left: w358 -> [w382]
                            shift-right: [w393] -> _
                            shift-left: _ -> [w381]
                            n87 = call-poly "ziGetValue.vi"("error in"=w381, "Path"="demods/0/sample", "Handle In"=w382) -> ("error out"=w387:errorcluster, "Demod Sample Out"=w385:T3, "Handle Out"=w388:T2)
                            n88 = Unbundle By Name(w385) -> ("X (Vrms)"=w384:dbl, "Y (Vrms)"=w383:dbl)  [unwired: 1 out]
                            n89 = call-poly "ziGetValue.vi"("error in"=w387, "Path"="demods/2/sample", "Handle In"=w388) -> ("error out"=w393:errorcluster, "Demod Sample Out"=w391:T3, "Handle Out"=w394:T2)
                            n90 = Unbundle By Name(w391) -> ("X (Vrms)"=w390:dbl, "Y (Vrms)"=w389:dbl)  [unwired: 1 out]
                          }
                          n91 = call "430_TCP_Query.vi"("Command"="FIELD:MAGnet?" ("String"), "connection ID"=w370) -> ("Response"=w369:string, "connection ID out"=w368:refnum<k5>)  [unwired: 5 in, 3 out]
                          n92 = call "430_TCP_Query.vi"("Command"="FIELD:MAGnet?" ("String"), "connection ID"=w374) -> ("Response"=w376:string, "connection ID out"=w373:refnum<k5>)  [unwired: 5 in, 3 out]
                          n93 = Fract/Exp String To Number(string=w369) -> (number=w359:dbl)  [unwired: 3 in, 1 out]
                          "Sweeping Magnetic Field (T)" <- w359
                          n94 = Fract/Exp String To Number(string=w376) -> (number=w372:dbl)  [unwired: 3 in, 1 out]
                          "Stable Magnetic Field (T)" <- w372
                          n95 = call "Array averaging_PK.vi"("Number averaging"="Number average", "numeric array"=w367) -> ("Average value"=w366:dbl)  [unwired: 9 in]
                          n96 = call "Array averaging_PK.vi"("Number averaging"="Number average", "numeric array"=w365) -> ("Average value"=w361:dbl)  [unwired: 9 in]
                          n97 = call "Array averaging_PK.vi"("Number averaging"="Number average", "numeric array"=w364) -> ("Average value"=w363:dbl)  [unwired: 9 in]
                          n98 = call "Array averaging_PK.vi"("Number averaging"="Number average", "numeric array"=w362) -> ("Average value"=w360:dbl)  [unwired: 9 in]
                          n99 = call "Array averaging_PK.vi"("Number averaging"="Number average", "numeric array"=w356) -> ("Average value"=w352:dbl)  [unwired: 9 in]
                          n100 = call "Array averaging_PK.vi"("Number averaging"="Number average", "numeric array"=w354) -> ("Average value"=w350:dbl)  [unwired: 9 in]
                          n101 = call "Array averaging_PK.vi"("Number averaging"="Number average", "numeric array"=w355) -> ("Average value"=w351:dbl)  [unwired: 9 in]
                          n102 = call "Array averaging_PK.vi"("Number averaging"="Number average", "numeric array"=w353) -> ("Average value"=w349:dbl)  [unwired: 9 in]
                        }
                      }
                      n103 = Subtract(x=w344, y=w343) -> (x-y=w342:u32)
                      n104 = Divide(x=w342, y=1000) -> (x/y=→"Time (s)":dbl)
                      n105 = local read "Sweeping Magnetic Field (T)"() -> (w312:dbl)
                      n106 = local read "Stable Magnetic Field (T)"() -> (w319:dbl)
                      n107 = local read "Time (s)"() -> (w318:dbl)
                      n108 = Divide(x=w325, y=w323) -> (x/y=w321:dbl)
                      "Rx 1 (ohm)" <- w321
                      n109 = Divide(x=w314, y=w313) -> (x/y=w311:dbl)
                      "Rx 2 (ohm)" <- w311
                      n110 = Bundle(w326, w321) -> (w347:cluster{dbl, dbl})  [unwired: 1 in]
                      n111 = Build Array(w319, w312, w318, w325, w324, w323, w322, w321) -> (w331:dbl[])
                      "data" <- w331
                      n112 = Bundle("Sweeping Magnetic Field (T)"=w312, w311) -> (w315:cluster{"Sweeping Magnetic Field (T)":dbl, dbl})  [unwired: 1 in]
                      n113 = Build Array(w319, w312, w318, w314, w317, w313, w316, w311) -> (w305:dbl[])
                      "data 2" <- w305
                      n114 = Build Array (concatenate)(w346, w347) -> (w345:cluster{dbl, "Field Reading":dbl}[])
                      "Rx vs H sweep (Device 1)" <- w345
                      n115 = Build Array (concatenate)(w308, w315) -> (w309:T4)
                      "Rx vs H sweep (Device 2)" <- w309
                      n116 = local read "File path 1"() -> (w333:path)
                      n117 = local read "File path 2"() -> (w304:path)
                      n118 = Array To Spreadsheet String(array=w331, 3:"%e" ("format string")) -> (spreadsheet string=w334:string)  [unwired: 1 in]
                      n119 = Array To Spreadsheet String(array=w305, 3:"%e" ("format string")) -> (spreadsheet string=w307:string)  [unwired: 1 in]
                      n120 = call <vilib>:"Write Characters To File.vi"("append to file? (new file:F)"=TRUE, "character string"=w334, "file path (dialog if empty)"=w333) -> ()  [unwired: 2 in, 1 out]
                      n121 = call <vilib>:"Write Characters To File.vi"("append to file? (new file:F)"=TRUE, "character string"=w307, "file path (dialog if empty)"=w304) -> ()  [unwired: 2 in, 1 out]
                      "Ix 1 (A)" <- w323
                      "Vx 1 (V)" <- w325
                      "Vy 1 (V)" <- w324
                      "Iy 1 (A)" <- w322
                      "Vx 2 (V)" <- w314
                      "Vy 2 (V)" <- w317
                      "Ix 2 (A)" <- w313
                      "Iy 2 (A)" <- w316
                    }
                  }
                }
              }
              n122 = call "430_TCP_Close.vi"("connection ID"=w221) -> ()  [unwired: 1 in, 2 out]
              n123 = call "ziClose.vi"("Handle In"=w223) -> ("Handle Out"=w206:T2)  [unwired: 1 in, 3 out]
              n124 = call "ziClose.vi"("Handle In"=w212) -> ("Handle Out"=w205:T2)  [unwired: 1 in, 3 out]
            }
          }
        }
      }
      n125 = call "430_TCP_Close.vi"("connection ID"=w97) -> ()  [unwired: 1 in, 2 out]
      n126 = Unbundle By Name(w100) -> ("status"=w99:bool)
      n127 = Or(x=w99, y="stop") -> ()  [unwired: 1 out]
    }
  }
